vi "S_SetProperty.vi"(0 "reference in":refnum<class "SubTemplate.lvclass">, 1 "Property":dbl, 5 "error in (no error)":errorcluster) -> (14 "reference out":refnum<class "SubTemplate.lvclass">, 19 "error out":errorcluster)   [LabVIEW 2020]
uses:
  <resource>/Framework/Providers/Open_GDS/ClassProviders/Provider_EndevoGOOP300/Templates/SubTemplate/SubTemplate.lvclass
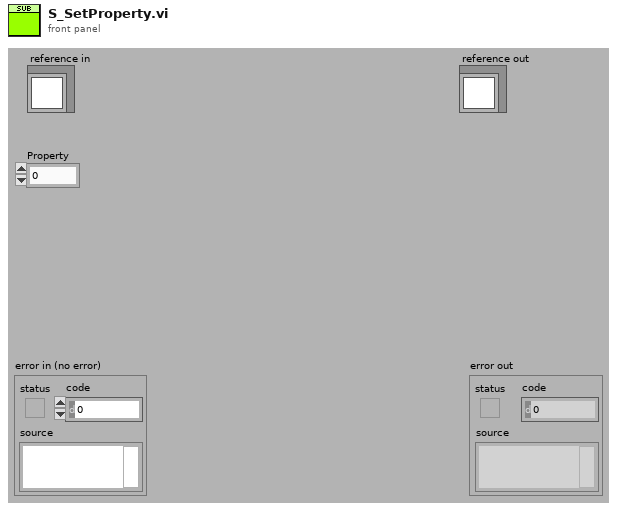
[diagram p1: front panel]
types:
  T1 = typedef "SubTemplate.lvclass/ObjectAttributes.ctl" = cluster{"Base class":T2}
  T2 = typedef "BaseTemplate.lvclass/ObjectAttributes.ctl" = cluster{"Attribute1":dbl}
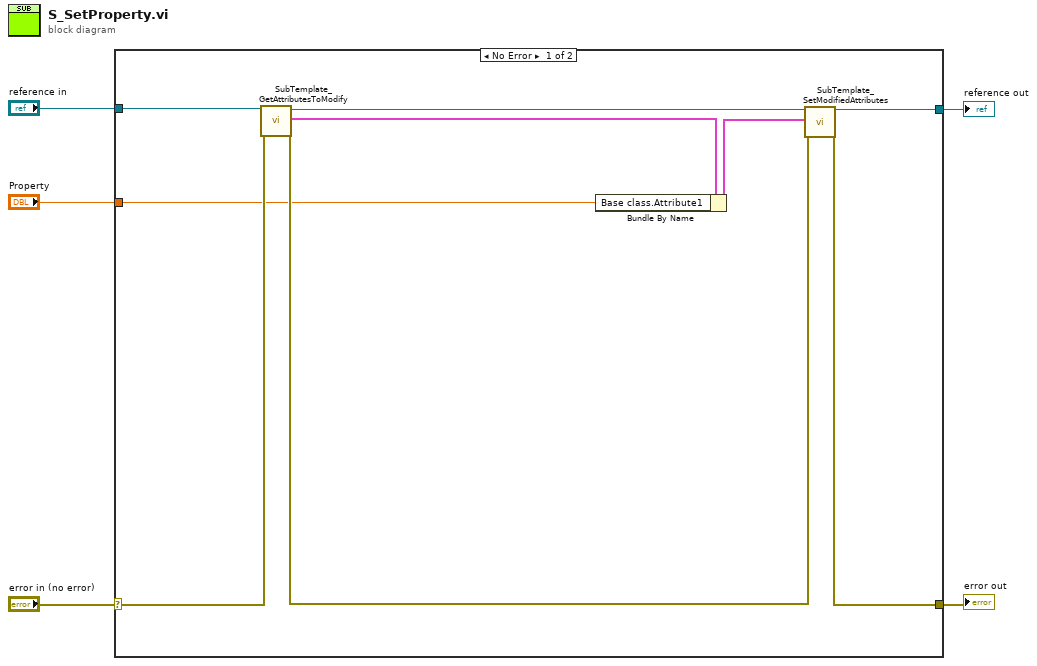
[diagram p0: block diagram]
diagram:
  n1 = case shown="No Error" "error in (no error)" {
    selector: "error in (no error)" -> [w9 w16]
    tunnel: [w11 w16] -> w4
    tunnel: [w8 w15] -> w2
    tunnel: "reference in" -> [w10 w15]
    tunnel: "Property" -> [w6 _]
    frame No Error {
      n2 = call <resource>:"SubTemplate_GetAttributesToModify.vi"("reference in"=w10, "error in (no error)"=w9) -> ("reference out"=w12:refnum<class "SubTemplate.lvclass">, "Attributes"=w14:T1, "error out"=w7:errorcluster)  [unwired: 14 in, 1 out]
      n3 = Bundle By Name(cluster=w14, "Base class.Attribute1"=w6) -> (w13:T1)
      n4 = call <resource>:"SubTemplate_SetModifiedAttributes.vi"("reference in"=w12, "Attributes"=w13, "error in (no error)"=w7) -> ("reference out"=w8:refnum<class "SubTemplate.lvclass">, "error out"=w11:errorcluster)  [unwired: 15 in]
    }
    frame Error {
    }
  }
  "error out" <- w4
  "reference out" <- w2
